vi "Inline vims in Library.vi"(7 "Just Fixup":bool, 8 "error in":errorcluster, 11 "Library":refnum<vi>) -> (0 "error out":errorcluster)   [LabVIEW 2020, in "vim-liner.lvlib"]
uses:
  vim-liner.lvlib
  <vilib>/Utility/traverseref.llb/TRef TravTarget.ctl
  9f827e63-bb42-40f9-9ba4-15158c3f13a4.vi
  <vilib>/Utility/traverseref.llb/VI Scripting - Traverse.lvlib
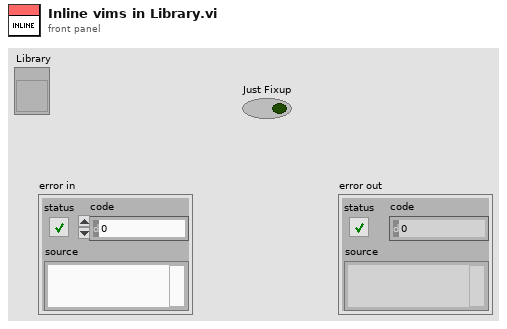
[diagram p1: front panel]
types:
  T1 = typedef "vim-liner.lvlib/vim-formation.ctl" = cluster{"ProjectItem Refnum":refnum<vi>, "Library Access Scope":enum32{"invalid scope", "public", "private", "protected", "community"}, "Library Qualified Name":string, "Path":path}
  T2 = typedef "TRef TravTarget.ctl" = enum16{"FP", "BD", "Other"}
  T3 = enum32{"invalid scope", "public", "private", "protected", "community"}
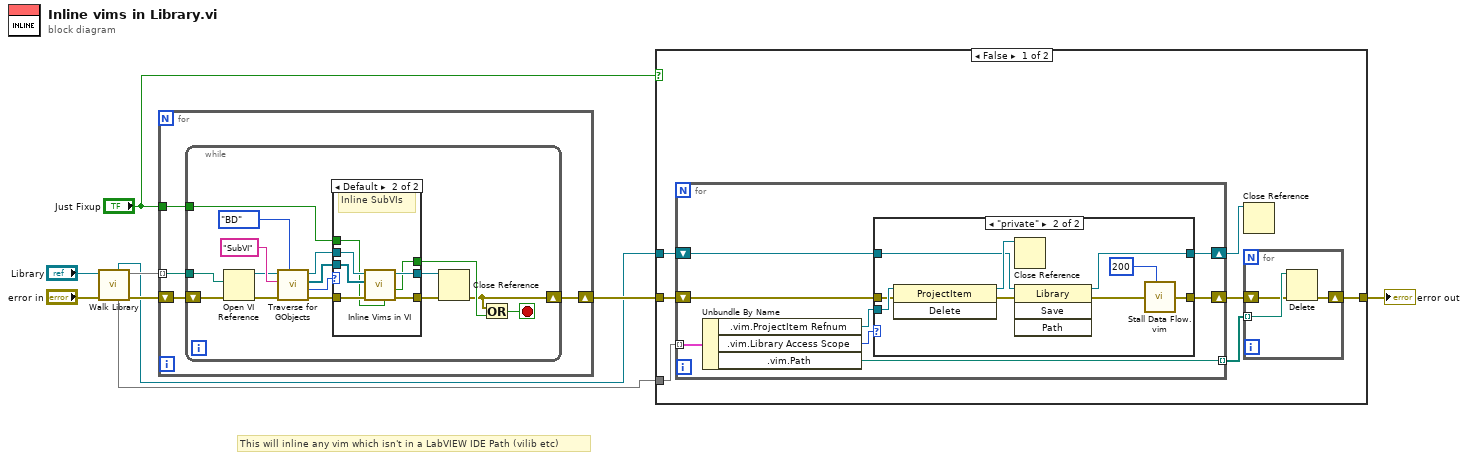
[diagram p0: block diagram]
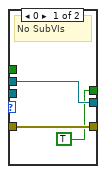
[diagram p4: hidden frame]
diagram:
  # "This will inline any vim which isn't in a LabVIEW IDE Path (vilib etc)"
  n1 = call "Walk Library.vi"("error in (no error)"="error in", "Library"="Library") -> ("error out"=w8:errorcluster, "All VIs"=w7:set{path}, "Vimformation"=w6:map{path, T1}, "Library Out"=w4:refnum<vi>)  [unwired: 6 in]
  n2 = for {
    shift-right: [w11] -> w5
    shift-left: w8 -> [w13]
    tunnel: w7 -> [w12] mode=indexing
    tunnel: "Just Fixup" -> [w10]
    n3 = while {
      tunnel: w12 -> [w28]
      shift-right: [w15] -> w11
      shift-left: w13 -> [w29]
      tunnel: w10 -> [w14]
      stop <- w16 stop-if-true
      n4 = Open VI Reference(vi path=w28, error in (no error)=w29) -> (vi reference=w18:refnum<vi>, error out=w19:errorcluster)  [unwired: 4 in]
      n5 = call <vilib>:"Traverse for GObjects.vi"("Traverse Target"=TRef_TravTarget."BD", "error in (no error)"=w19, "Class Name"="SubVI", "VI Refnum"=w18) -> ("error out"=w24:errorcluster, "# of Refs"=w23:i32, "References"=w20:refnum<vi>[], "dup VI Refnum"=w25:refnum<vi>)  [unwired: 4 in]
      n6 = case shown="Default" w23 {
        tunnel: w25 -> [w31 w39]
        tunnel: w24 -> [w32 w38]
        tunnel: [w32 w36] -> w22
        tunnel: [w31 w37] -> w21
        tunnel: w20 -> [_ w35]
        tunnel: [TRUE ("Nothing to Inline") w34] -> w17
        tunnel: w14 -> [_ w33]
        frame 0 {
          # "No SubVIs"
        }
        frame Default {
          # "Inline SubVIs"
          n7 = call "Inline Vims in VI.vi"("Just Fixup"=w33, "error in (no error)"=w38, "References"=w35, "VI in"=w39) -> ("error out"=w36:errorcluster, "Nothing to Inline"=w34:bool, "VI out"=w37:refnum<vi>)  [unwired: 5 in]
        }
      }
      n8 = Close Reference(reference=w21, error in (no error)=w22) -> (error out=w15:errorcluster)
      n9 = Or(x=w15, y=w17) -> (x .or. y?=w16:bool)
    }
  }
  n10 = case shown="False" "Just Fixup" {
    tunnel: w6 -> [w46 _]
    tunnel: w5 -> [w45 w69]
    tunnel: w4 -> [w41 _]
    tunnel: [w42 w69] -> w3
    frame False {
      n11 = for {
        tunnel: w46 -> [w50] mode=indexing
        shift-right: [w54] -> w44
        shift-left: w45 -> [w55]
        tunnel: [w53] -> w43 mode=indexing
        shift-right: [w51] -> w40
        shift-left: w41 -> [w52]
        n12 = Unbundle By Name(w50) -> (".vim.ProjectItem Refnum"=w56:refnum<vi>, ".vim.Library Access Scope"=w57:T3, ".vim.Path"=w53:path)
        n13 = case shown="\"private\"" w57 {
          tunnel: w56 -> [_ w68]
          tunnel: w55 -> [w59 w67]
          tunnel: [w59 w63] -> w54
          tunnel: w52 -> [w58 w61]
          tunnel: [w58 w60] -> w51
          frame Default {
          }
          frame "private" {
            n14 = invoke class="ProjectItem" method="Delete"(reference=w68, error in=w67) -> (reference out=w66:refnum<vi>, error out=w65:errorcluster)  [unwired: 1 in, 1 out]
            n15 = Close Reference(reference=w66) -> ()  [unwired: 1 in, 1 out]
            n16 = invoke class="Library" method="Save"(reference=w61, error in=w65) -> (reference out=w60:refnum<vi>, error out=w64:errorcluster)  [unwired: 2 in, 2 out]
            n17 = call "Stall Data Flow.vim"("value in"=w64, "milliseconds to wait"=u32 200) -> ("value out"=w63:errorcluster)  [unwired: 1 out]
          }
        }
      }
      n18 = Close Reference(reference=w40) -> ()  [unwired: 1 in, 1 out]
      n19 = for {
        tunnel: w43 -> [w49] mode=indexing
        shift-right: [w47] -> w42
        shift-left: w44 -> [w48]
        n20 = Delete(path (use dialog)=w49, error in=w48) -> (error out=w47:errorcluster)  [unwired: 3 in, 2 out]
      }
    }
    frame True {
    }
  }
  "error out" <- w3
